vi "ILYA_ADQ_GetData.vi"(5 "buffer_chB_in":i16[](array[numeric]), 7 "buffer_chA_in":i16[](array[numeric]), 8 "error in":errorcluster, 9 "number_of_records":u32, 10 "samples_per_record":u32, 11 "adq_cu_ptr":u32) -> (0 "error out":errorcluster, 2 "function return":i32, 3 "adq_cu_ptr":u32, 4 "buffer_chB_out":i16[](array[numeric]), 6 "buffer_chA_out":i16[](array[numeric]))   [LabVIEW 2013]
uses:
  GetData_DLL.dll
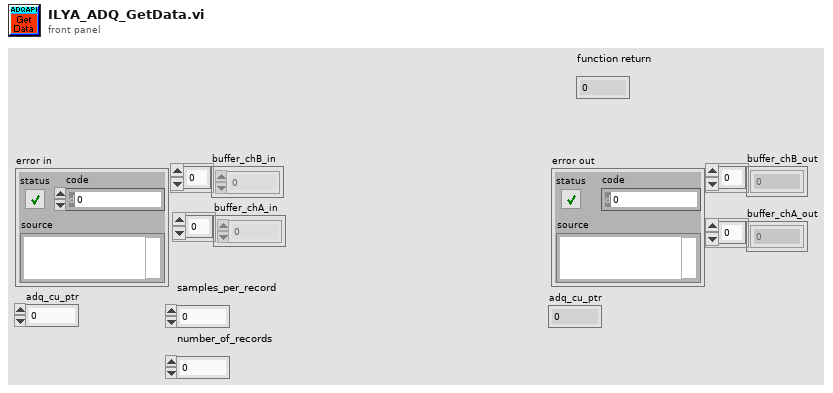
[diagram p1: front panel]
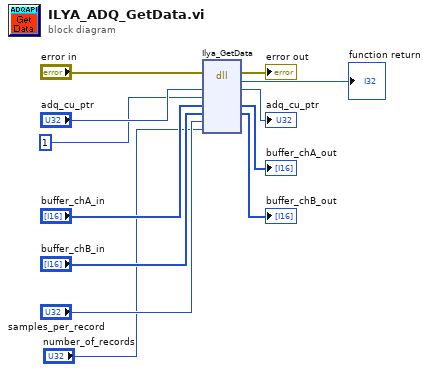
[diagram p0: block diagram]
diagram:
  n1 = dll-call lib="C:/Users/astafiev/Desktop/IlyaDrive/@photonCounting/LabView_Imperium/GetData_DLL.dll" fn="Ilya_GetData"(error in="error in", "adq_cu_ptr"="adq_cu_ptr", "adq_num"=1, "buffer_chA"="buffer_chA_in", "buffer_chB"="buffer_chB_in", "samples_per_record"="samples_per_record", "number_of_records"="number_of_records") -> (error out=→"error out":errorcluster, "return type"=→"function return":i32, "adq_cu_ptr"=→"adq_cu_ptr":u32, "buffer_chA"=→"buffer_chA_out":i16[], "buffer_chB"=→"buffer_chB_out":i16[])  [unwired: 5 in, 1 out]
